vi "Main.vi"() -> ()   [LabVIEW 2019]
uses:
  <vilib>/MakerHub/LINX/LMH-LINX.lvlib
panel:
  out "WFS1 Chart":waveform(dbl)[](graph)
  out "WFS1":dbl format="%.2g"
  out "M1 Chart":waveform(dbl)[](graph)
  out "M2 Chart":waveform(dbl)[](graph)
  out "M4 Chart":waveform(dbl)[](graph)
  out "M3 Chart":waveform(dbl)[](graph)
  in  "VISA":refnum<visa-resource-name>="COM25"
  out "M4":dbl format="%.2g"
  out "M3":dbl format="%.2g"
  in  "Readout Interval (ms)":i32=1000
  out "M2":dbl format="%.2g"
  out "M1":dbl format="%.2g"
  out "Readout Status":bool
  out "Last Measured":timestamp format="%<%Y-%m-%d %H:%M:%S>T"
  in  "Stop":bool
  # "LCW Flow Monitor"
  # "GPM"
  # "GPM"
  # "GPM"
  # "GPM"
  # "GPM"
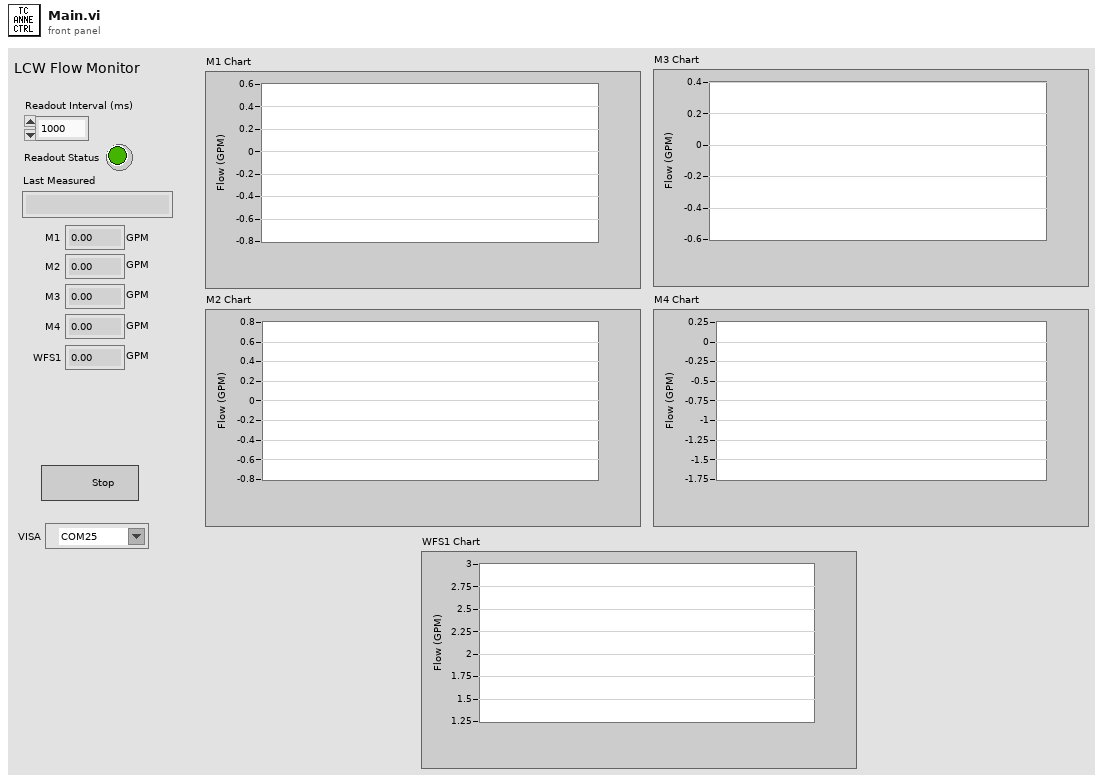
[diagram p1: front panel]
types:
  T1 = typedef "LMH-LINX.lvlib/LINX Ref.ctl" = cluster{"IO":T2, "Interface":T3, "LINX Device Config":T4}
  T2 = typedef "LMH-LINX.lvlib/Platform.ctl" = enum16{"Remote", "Local"}
  T3 = typedef "LMH-LINX.lvlib/Interface.ctl" = enum16{"Serial", "TCP"}
  T4 = typedef "LMH-LINX.lvlib/Device.lvlib/LINX Device Config.ctl" = cluster{"Interface":T3, "COM Port":refnum<visa-resource-name>, "TCP Configuration":T5, "Device Family":u8, "Device ID":u8, "Device Name":string, "TCP Ref":refnum<k5>, "Channels":T6}
  T5 = typedef "LMH-LINX.lvlib/Device.lvlib/TCP Config.ctl" = cluster{"IP Address":string, "Port":u16}
  T6 = typedef "LMH-LINX.lvlib/Channels.ctl" = cluster{"DI":u8[], "DO":u8[], "AI":u8[], "AO":u8[], "PWM":u8[], "QE":u8[], "UART":u8[], "I2C 2":u8[], "SPI":u8[], "CAN":u8[], "Servo":u8[], "AI Ref (V)":dbl, "AI Resolution (Bits)":u8, "AO Ref (V)":dbl, "AO Resolution (Bits)":u8}
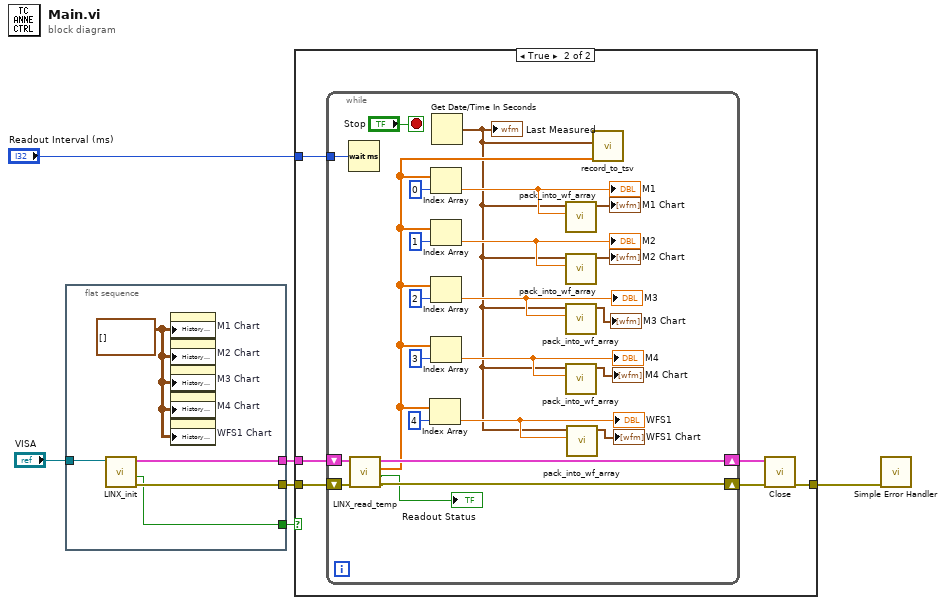
[diagram p0: block diagram]
diagram:
  n1 = flat-sequence {
    tunnel: [w8] -> w4
    tunnel: [w11] -> w3
    tunnel: "VISA" -> [w10]
    tunnel: [w9] -> w1
    frame #0 {
      w7 = waveform(dbl)[][] [] ("History Data")
      n2 = call "LINX_init.vi"("VISA"=w10) -> ("error out"=w11:errorcluster, "status"=w8:bool, "LINX Resource"=w9:T1)  [unwired: 8 in]
      n3 = property on="M1 Chart" class="WFChart (strict)"("History Data"=w7) -> ()  [unwired: 2 in, 2 out]
      n4 = property on="M2 Chart" class="WFChart (strict)"("History Data"=w7) -> ()  [unwired: 2 in, 2 out]
      n5 = property on="M3 Chart" class="WFChart (strict)"("History Data"=w7) -> ()  [unwired: 2 in, 2 out]
      n6 = property on="M4 Chart" class="WFChart (strict)"("History Data"=w7) -> ()  [unwired: 2 in, 2 out]
      n7 = property on="WFS1 Chart" class="WFChart (strict)"("History Data"=w7) -> ()  [unwired: 2 in, 2 out]
    }
  }
  n8 = case shown="True" w4 {
    tunnel: "Readout Interval (ms)" -> [_ w18]
    tunnel: [w12 w15] -> w5
    tunnel: w3 -> [w12 w17]
    tunnel: w1 -> [_ w16]
    frame False {
    }
    frame True {
      n9 = while {
        shift-right: [w25] -> w14
        shift-left: w17 -> [w28]
        tunnel: w18 -> [w39]
        shift-right: [w26] -> w13
        shift-left: w16 -> [w27]
        stop <- "Stop" stop-if-true
        n10 = Wait (ms)(milliseconds to wait=w39) -> ()  [unwired: 1 out]
        n11 = call "LINX_read_temp.vi"("Error In"=w28, "LINX Resource"=w27) -> ("Error Out"=w25:errorcluster, "status"=→"Readout Status":bool, "array_flow"=w20:dbl[], "LINX Resource Out"=w26:T1)  [unwired: 6 in]
        n12 = Index Array(array=w20, index=4) -> (element=w21:dbl)
        "WFS1" <- w21
        n13 = Index Array(array=w20, index=0) -> (element=w36:dbl)
        "M1" <- w36
        n14 = Index Array(array=w20, index=1) -> (element=w35:dbl)
        "M2" <- w35
        n15 = Index Array(array=w20, index=2) -> (element=w30:dbl)
        "M3" <- w30
        n16 = Index Array(array=w20, index=3) -> (element=w29:dbl)
        "M4" <- w29
        n17 = Get Date/Time In Seconds() -> (seconds since 1Jan1904=w19:timestamp)
        "Last Measured" <- w19
        n18 = call "pack_into_wf_array.vi"("value"=w36, "time"=w19) -> ("waveform_array"=→"M1 Chart":waveform(dbl)[])  [unwired: 9 in]
        n19 = call "pack_into_wf_array.vi"("value"=w35, "time"=w19) -> ("waveform_array"=→"M2 Chart":waveform(dbl)[])  [unwired: 9 in]
        n20 = call "pack_into_wf_array.vi"("value"=w30, "time"=w19) -> ("waveform_array"=→"M3 Chart":waveform(dbl)[])  [unwired: 9 in]
        n21 = call "pack_into_wf_array.vi"("value"=w29, "time"=w19) -> ("waveform_array"=→"M4 Chart":waveform(dbl)[])  [unwired: 9 in]
        n22 = call "pack_into_wf_array.vi"("value"=w21, "time"=w19) -> ("waveform_array"=→"WFS1 Chart":waveform(dbl)[])  [unwired: 9 in]
        n23 = call "record_to_tsv.vi"("temperatures"=w20, "time"=w19) -> ()  [unwired: 10 in]
      }
      n24 = call <vilib>:"Close.vi"("Error In"=w14, "LINX Resource"=w13) -> ("Error Out"=w15:errorcluster)  [unwired: 9 in]
    }
  }
  n25 = call <vilib>:"Simple Error Handler.vi"("error in (no error)"=w5) -> ()  [unwired: 4 in, 5 out]
